vi "Make Figure array.vi"(3 "Aantal hoekken (n)":dbl=5.0, 4 "Straal (s)":dbl=5.0, 5 "Speed":dbl=3.0) -> (0 "Figur array":dbl[][](array[numeric]), 1 "waypoints":dbl[][](array[numeric]), 2 "Route Array":dbl[][](array[numeric]))   [LabVIEW 2022 SP3]
panel:
  out "XY Graph 2":cluster{dbl[], dbl[]}[](graph)
  out "waypointsWOW":dbl[][](array[numeric])
  out "XY Graph":cluster{dbl[], dbl[]}[](graph)
  out "Array":dbl[][](array[numeric])
  out "hoek":dbl
  out "zijde":dbl
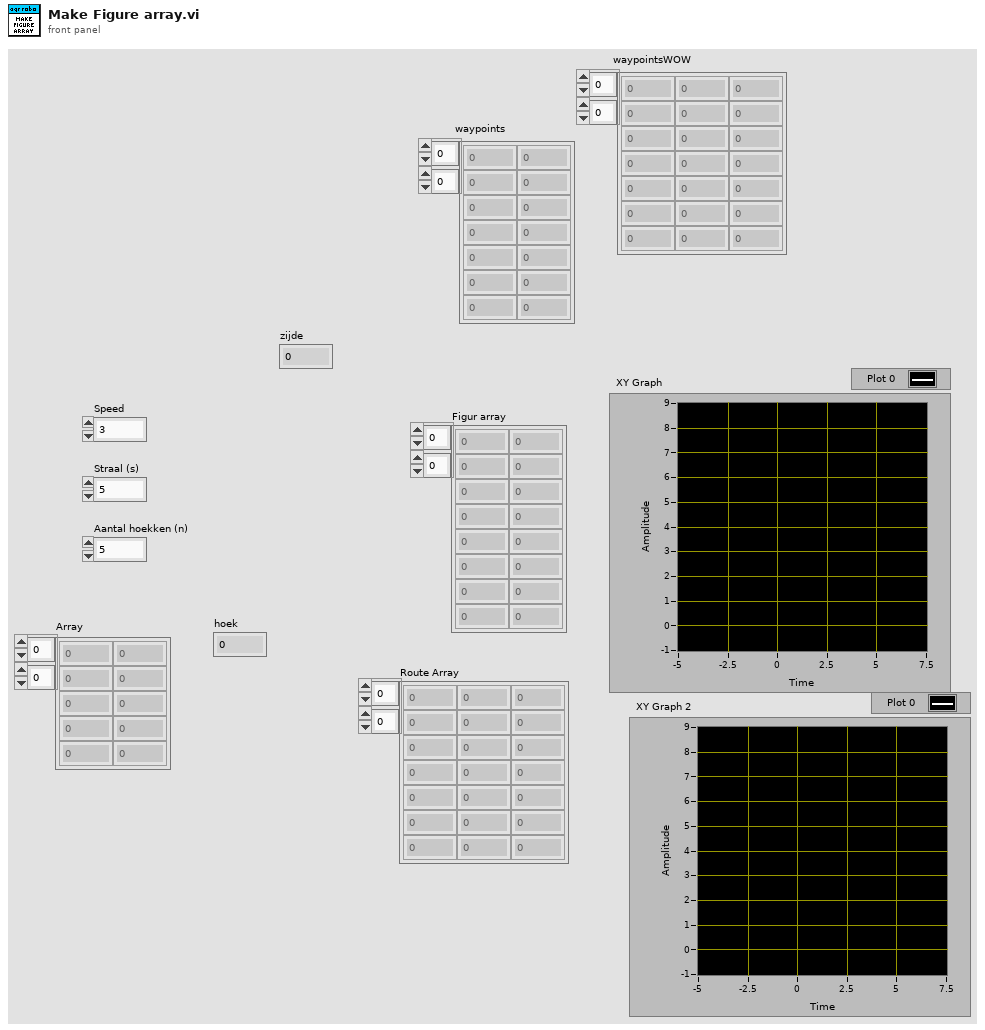
[diagram p1: front panel]
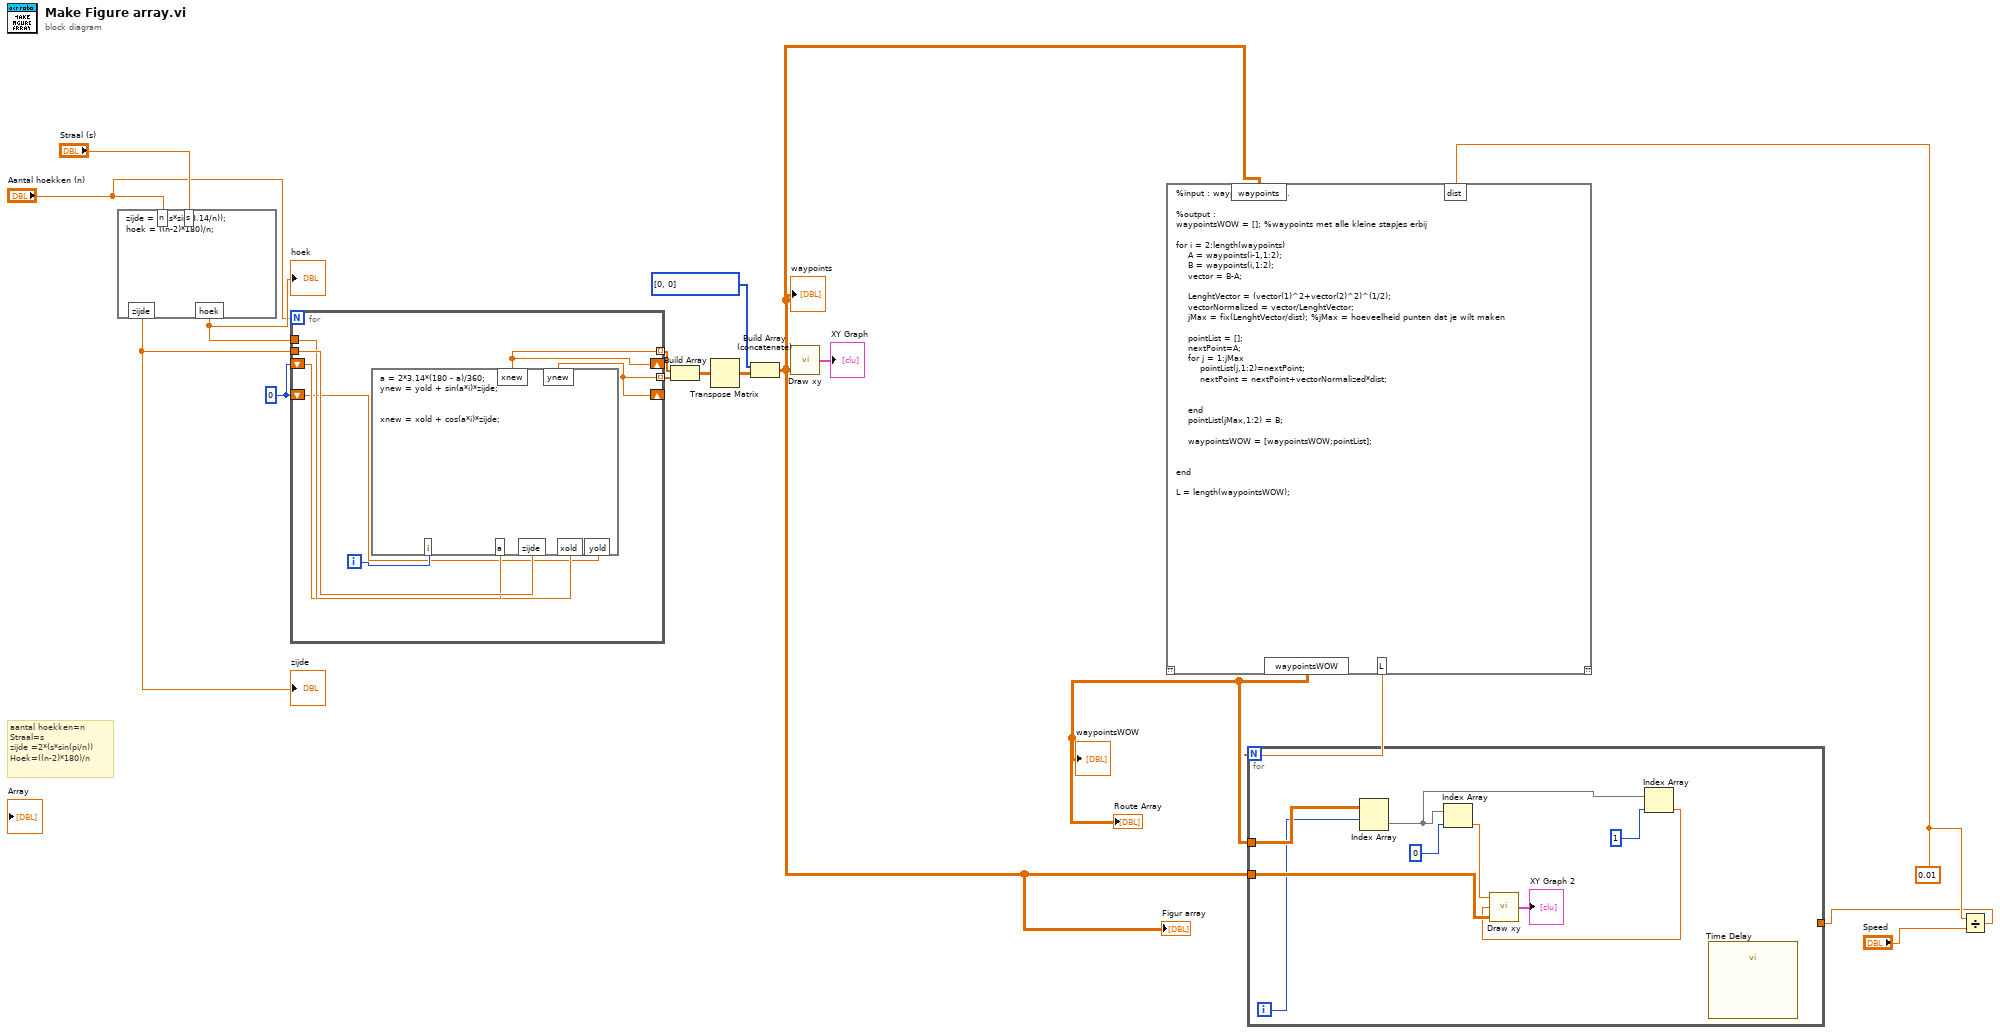
[diagram p0: block diagram]
diagram:
  w5 = 0.01
  w10 = 0
  # "aantal hoekken=n\nStraal=s\nzijde =2*(s*sin(pi/n))\nHoek=((n-2)*180)/n"
  n1 = formula code="zijde = 2*(s*sin(3.14/n));\nhoek = ((n-2)*180)/n;"("n"="Aantal hoekken (n)", "s"="Straal (s)") -> ("zijde"=w16:dbl, "hoek"=w15:dbl)
  "zijde" <- w16
  "hoek" <- w15
  n2 = for {
    N: "Aantal hoekken (n)" -> [_]
    tunnel: w16 -> [w23]
    tunnel: w15 -> [w22]
    shift-right: [w19] -> _
    shift-left: w10 -> [w21]
    shift-right: [w18] -> _
    shift-left: w10 -> [w20]
    tunnel: [w19] -> w13 mode=indexing
    tunnel: [w18] -> w12 mode=indexing
    i -> [w24]
    n3 = formula code="a = 2*3.14*(180 - a)/360;\nynew = yold + sin(a*i)*zijde;\n \n\nxnew = xold + cos(a*i)*zijde;"("i"=w24, "a"=w22, "zijde"=w23, "xold"=w21, "yold"=w20) -> ("xnew"=w19:dbl, "ynew"=w18:dbl)
  }
  n4 = Build Array(w13, w12) -> (w11:dbl[][])
  n5 = Transpose Matrix(1:w11) -> (0:w7:dbl[][])
  n6 = Build Array (concatenate)(i32[] [0, 0], w7) -> (w1:dbl[][])
  "Figur array" <- w1
  "waypoints" <- w1
  n7 = call "Draw xy.vi"("Figur array"=w1) -> ("XY Graph"=→"XY Graph":cluster{dbl[], dbl[]}[])  [unwired: 2 in]
  n8 = script code="%input : waypoints en dist..\n\n%output : \nwaypointsWOW = []; %waypoints met alle kleine stapjes erbij\n\nfor i = 2:length(waypoints)\n    A = waypoints(i-1,1:2);\n    B = waypoints(i,1:2);\n    vector = B-A;\n\n    LenghtVector = (vector(1)^2+vector(2)^2)^(1/2);\n    vectorNormalized = vector/LenghtVector;\n    jMax = fix(LenghtVector/dist); %jMax = hoeveelheid punten dat je wilt maken\n\n    pointList = [];\n    nextPoint=A;\n    for j = 1:jMax\n        pointList(j,1:2)=nextPoint;\n        nextPoint = nextPoint+vectorNormalized*dist;\n     \n\n    end\n    pointList(jMax,1:2) = B;\n\n    waypointsWOW = [waypointsWOW;pointList];\n\n\nend\n\nL = length(waypointsWOW);"("waypoints"=w1, "dist"=w5) -> ("waypointsWOW"=w2:dbl[][], "L"=w6:dbl)  [unwired: 1 in, 1 out]
  "Route Array" <- w2
  "waypointsWOW" <- w2
  n9 = Divide(x=w5, y="Speed") -> (x/y=w3:dbl)
  n10 = for {
    N: w6 -> [_]
    tunnel: w2 -> [w31]
    tunnel: w1 -> [w32]
    tunnel: w3 -> [_]
    i -> [w30]
    n11 = Index Array(array=w31, index (row)=w30) -> (element=w27:dbl[])  [unwired: 1 in]
    n12 = Index Array(array=w27, index=0) -> (element=w26:dbl)
    n13 = Index Array(array=w27, index=1) -> (element=w25:dbl)
    n14 = call "Draw xy.vi"("Figur array"=w32, "Y"=w25, "x"=w26) -> ("XY Graph"=→"XY Graph 2":cluster{dbl[], dbl[]}[])
    n15 = call "Time Delay"() -> ()  [unwired: 11 in, 1 out]
  }
